vi "PicoScope2000aExampleBlockAdvancedTrigger.vi"() -> ()   [LabVIEW 2010]
doc: "ps2000a API Block Capture example"
uses:
  shared/PicoBuffers.ctl
  <vilib>/Waveform/DWDTOps.llb/DWDT Analog to Digital.vi
  shared/Buffer and Transfer Settings.ctl
  shared/Acquisition Settings.ctl
  PicoScope2000aLib/PicoScope2000aAnalogChannelSettings.ctl
  PicoScope2000aLib/PicoScope2000aDigitalChannelSettings.ctl
panel:
  in  "roundFaster":bool=TRUE
  in  "timeIntervalRequested":dbl format="%#6_6p"
  in  "Write to TDMS":bool
  in  "Pulse Width Qualifier Settings":T1={"Direction"=2, "Lower Limit"=0, "Upper Limit"=0, "Pulse Width Type"=0} {"Pulse Width Type" items=["None", "Less Than", "Greater Than", "In Range", "Out of Range"]; "Direction" items=["Rising"=2, "Falling"=3]}
  in  "Pulse Width Qualifier Conditions":T2 {"Condition Logic" items=["AND", "OR", "XOR"]}
  in  "Auto Trigger (ms)":i32=1000
  in  "Channel A Trigger Properties":T3={"thresholdUpper"=0, "thresholdUpperHysteresis"=0, "thresholdLower"=0, "thresholdLowerHysteresis"=0, "Threshold Mode"=0, "Direction"=0, "Available"=TRUE} {"Direction" items=["Above / Inside", "Below / Outside", "Rising / Enter", "Falling / Exit", "Rising or Falling / Enter or Exit", "Above Lower", "Below Lower", "Rising Lower", "Falling Lower", "Positive Runt", "Negative Runt"]; "Threshold Mode" items=["Level", "Window"]}
  in  "Digital Port  0":T4 {"Direction Channel 7" items=["Don't Care", "Low", "High", "Rising", "Falling"]; "Direction Channel 6" items=["Don't Care", "Low", "High", "Rising", "Falling"]; "Direction Channel 5" items=["Don't Care", "Low", "High", "Rising", "Falling"]; "Direction Channel 4" items=["Don't Care", "Low", "High", "Rising", "Falling"]; "Direction Channel 3" items=["Don't Care", "Low", "High", "Rising", "Falling"]; "Direction Channel 2" items=["Don't Care", "Low", "High", "Rising", "Falling"]; "Direction Channel 1" items=["Don't Care", "Low", "High", "Rising", "Falling"]; "Direction Channel 0" items=["Don't Care", "Low", "High", "Rising", "Falling"]}
  in  "Trigger Conditions":T5 {"Condition Logic" items=["AND", "OR", "XOR"]}
  out "Properties Panel":T6 {"Max Total Capture Time Available (sec)" format="%.3p"; "Sample Frequency" format="%.3p"; "Sample Internal" format="%.3p"; "Max Samples Available" format="%.3p"; "Total Capture Time (sec)" format="%.3p"}
  in  "Port 0 Settings":T7={"Enabled"=FALSE, "Logic Level"=9830} {"Logic Level" items=["1.5V TTL"=9830, "2.5V CMOS"=16383]}
  in  "Channel A Settings":T8={"Enabled"=TRUE, "Coupling"=1, "Range"=6, "Analogue Offset"=0.0} {"Analogue Offset" format="%#_6p"; "Range" items=["20 mV"=1, "50 mV"=2, "100 mV"=3, "200 mV"=4, "500 mV"=5, "1 V"=6, "2 V"=7, "5 V"=8, "10 V"=9, "20 V"=10]; "Coupling" items=["AC", "DC"]}
  out "Device Info":T9={"Driver Version"="2.1.104.3324", "USB Version"="2.0", "Hardware"="1", "Variant"="2206A", "Batch and Serial"="CV676/049", "Cal Date"="19Sep17", "Kernel Version"="1.0", "Digital HW Version"="1", "Analogue HW Version"="1", "Firmware 1"="1.3.3.0", "Firmware 2"="0.5.47.0", "MSO"=FALSE, "Number of Channels"=2}
  out "overflow":i16 format="%06b"
  in  "Apply Settings":bool
  out "error out":errorcluster
  in  "Data file":path=path "PicoScope2000aExampleAdvancedTrgger Data"
  in  "Buffer and Transfer Settings":T10={"startIndex"=0, "Samples"=32000, "Down Sample Ratio"=1, "Down-Sample Mode"=0} {"Down-Sample Mode" items=["RAW none"=2147483648, "None"=0, "Aggregate"=1, "Decimate"=2, "Average"=4]; "Down Sample Ratio" step=1; "Samples" format="%_6p"}
  in  "Acquisition Settings":T11={"preTriggerSamples"=0, "postTriggerSamples"=32000, "timebase"=0} {"postTriggerSamples" format="%_6p"; "preTriggerSamples" format="%_6p"}
  out "Port 0":digitalwaveform(graph)={"t0"=timestamp(0 s since 1904-01-01), "dt"=8e-09, "Y"={"transitions"=[], "data"=[]}}
  in  "stop":bool
  out "Analog Channels":cluster{i32, sgl, "Data":dbl[]}[](graph)
  in  "Serial Number":string
  in  "Use Serial Number":bool
  in  "error in (no error)":errorcluster
  # "Bit 0 = ChA"
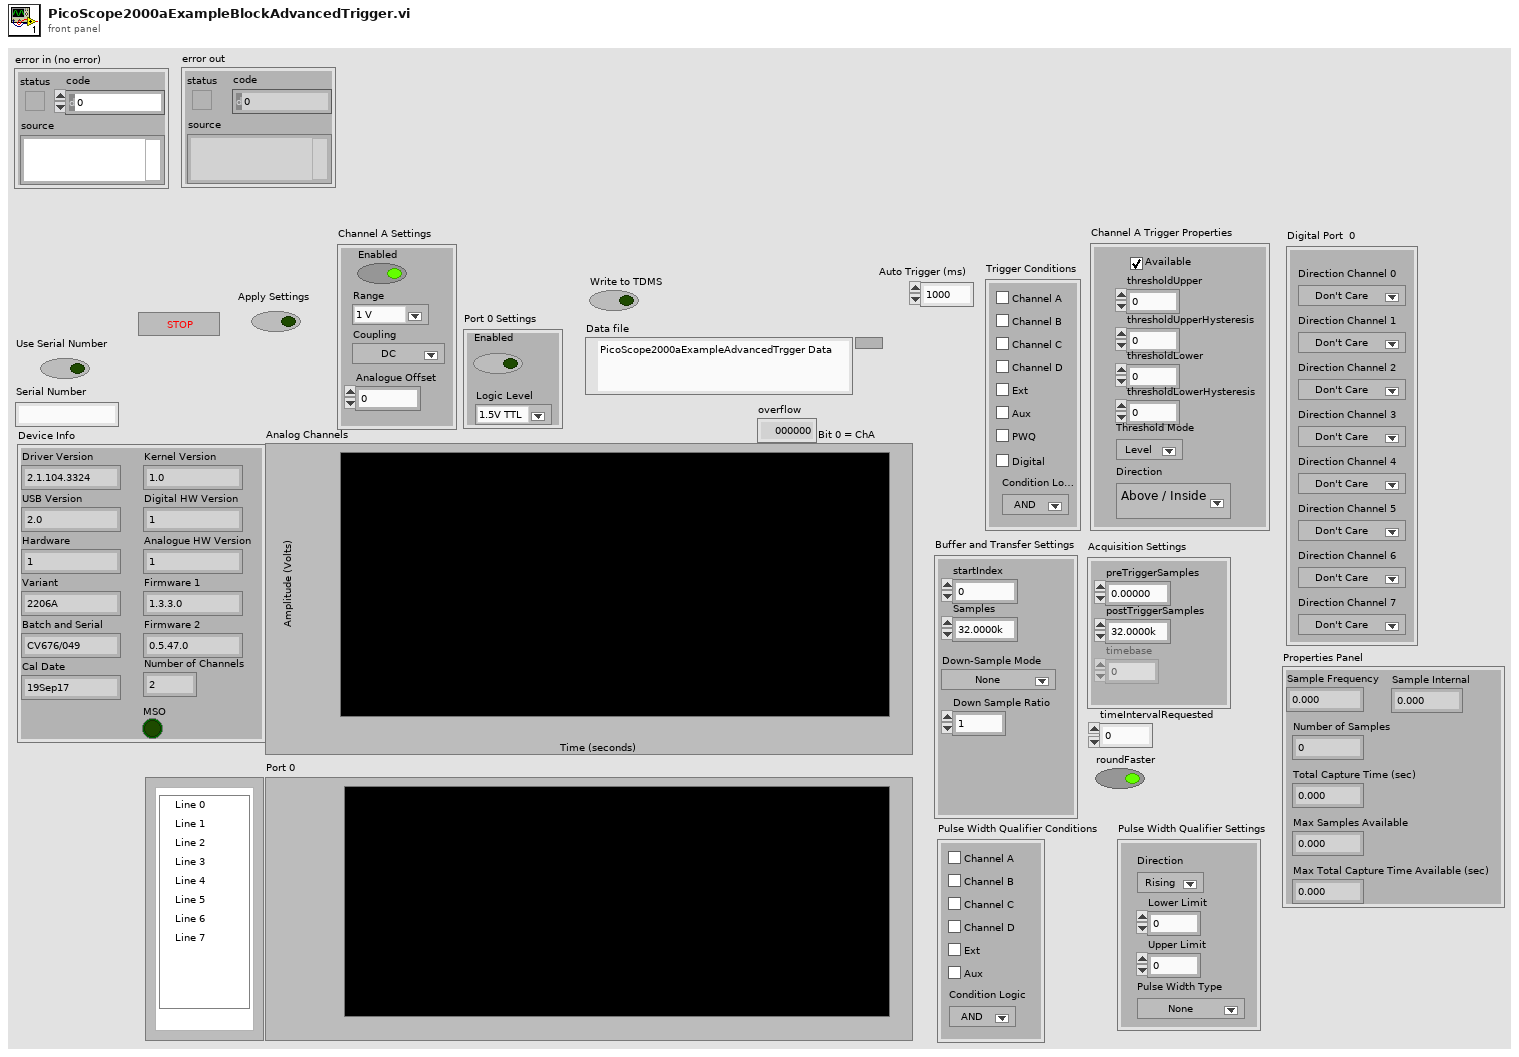
[diagram p1: front panel]
types:
  T1 = cluster{"Direction":i32, "Lower Limit":u32, "Upper Limit":u32, "Pulse Width Type":i32}
  T2 = cluster{"Channel A":bool, "Channel B":bool, "Channel C":bool, "Channel D":bool, "Aux":bool, "Condition Logic":u16, "Ext":bool}
  T3 = cluster{"thresholdUpper":i16, "thresholdUpperHysteresis":u16, "thresholdLower":i16, "thresholdLowerHysteresis":u16, "Threshold Mode":i32, "Direction":i32, "Available":bool}
  T4 = cluster{"Direction Channel 0":u16, "Direction Channel 1":u16, "Direction Channel 2":u16, "Direction Channel 3":u16, "Direction Channel 4":u16, "Direction Channel 5":u16, "Direction Channel 6":u16, "Direction Channel 7":u16}
  T5 = cluster{"Channel A":bool, "Channel B":bool, "Channel C":bool, "Channel D":bool, "Aux":bool, "PWQ":bool, "Condition Logic":u16, "Ext":bool, "Digital":bool}
  T6 = cluster{"Sample Frequency":sgl, "Sample Internal":sgl, "Max Samples Available":i32, "Number of Samples":u32, "Total Capture Time (sec) ":sgl, "Max Total Capture Time Available (sec)":sgl}
  T7 = typedef "PicoScope2000aDigitalChannelSettings.ctl" = cluster{"Enabled":bool, "Logic Level":i16}
  T8 = typedef "PicoScope2000aAnalogChannelSettings.ctl" = cluster{"Enabled":bool, "Coupling":i16, "Range":u32, "Analogue Offset":sgl}
  T9 = cluster{"Driver Version":string, "USB Version":string, "Hardware":string, "Variant":string, "Batch and Serial":string, "Cal Date":string, "Kernel Version":string, "Digital HW Version":string, "Analogue HW Version":string, "Firmware 1":string, "Firmware 2":string, "MSO":bool, "Number of Channels":i16}
  T10 = typedef "Buffer and Transfer Settings.ctl" = cluster{"startIndex":u64, "Samples":u64, "Down Sample Ratio":u64, "Down-Sample Mode":u32}
  T11 = typedef "Acquisition Settings.ctl" = cluster{"preTriggerSamples":u64, "postTriggerSamples":u64, "timebase":u32}
  T12 = typedef "PicoBuffers.ctl" = cluster{"Max Buffer Pointers":u64[][][], "Min Buffer Pointers":u64[][][], "StreamingDataInfo":cluster{"Channel":u32, "Down-Sample Mode":u32, "PICO_DATA_TYPE":enum32{"PICO_INT8_T", "PICO_INT16_T", "PICO_INT32_T", "PICO_UINT32_T", "PICO_INT64_T", ""}, "Samples":i32, "bufferIndex":u64, "startIndex":i32, "overflow":i16}[][]}
  T13 = enum16{"open", "open or create", "create or replace", "create", "open (read-only)"}
  T14 = cluster{"Channel A Buffer":i16[], "Channel B Buffer":i16[], "Channel C Buffer":i16[], "Channel D Buffer":i16[], "Channel E Buffer":i16[], "Channel F Buffer":i16[], "Channel G Buffer":i16[], "Channel H Buffer":i16[], "Port 0 Buffer":i16[], "Port 1 Buffer":i16[]}[]
  T15 = cluster{"Channel A Buffer":i16[], "Channel B Buffer":i16[], "Channel C Buffer":i16[], "Channel D Buffer":i16[], "Channel E Buffer":i16[], "Channel F Buffer":i16[], "Channel G Buffer":i16[], "Channel H Buffer":i16[], "Port 0 Buffer":i16[], "Port 1 Buffer":i16[]}
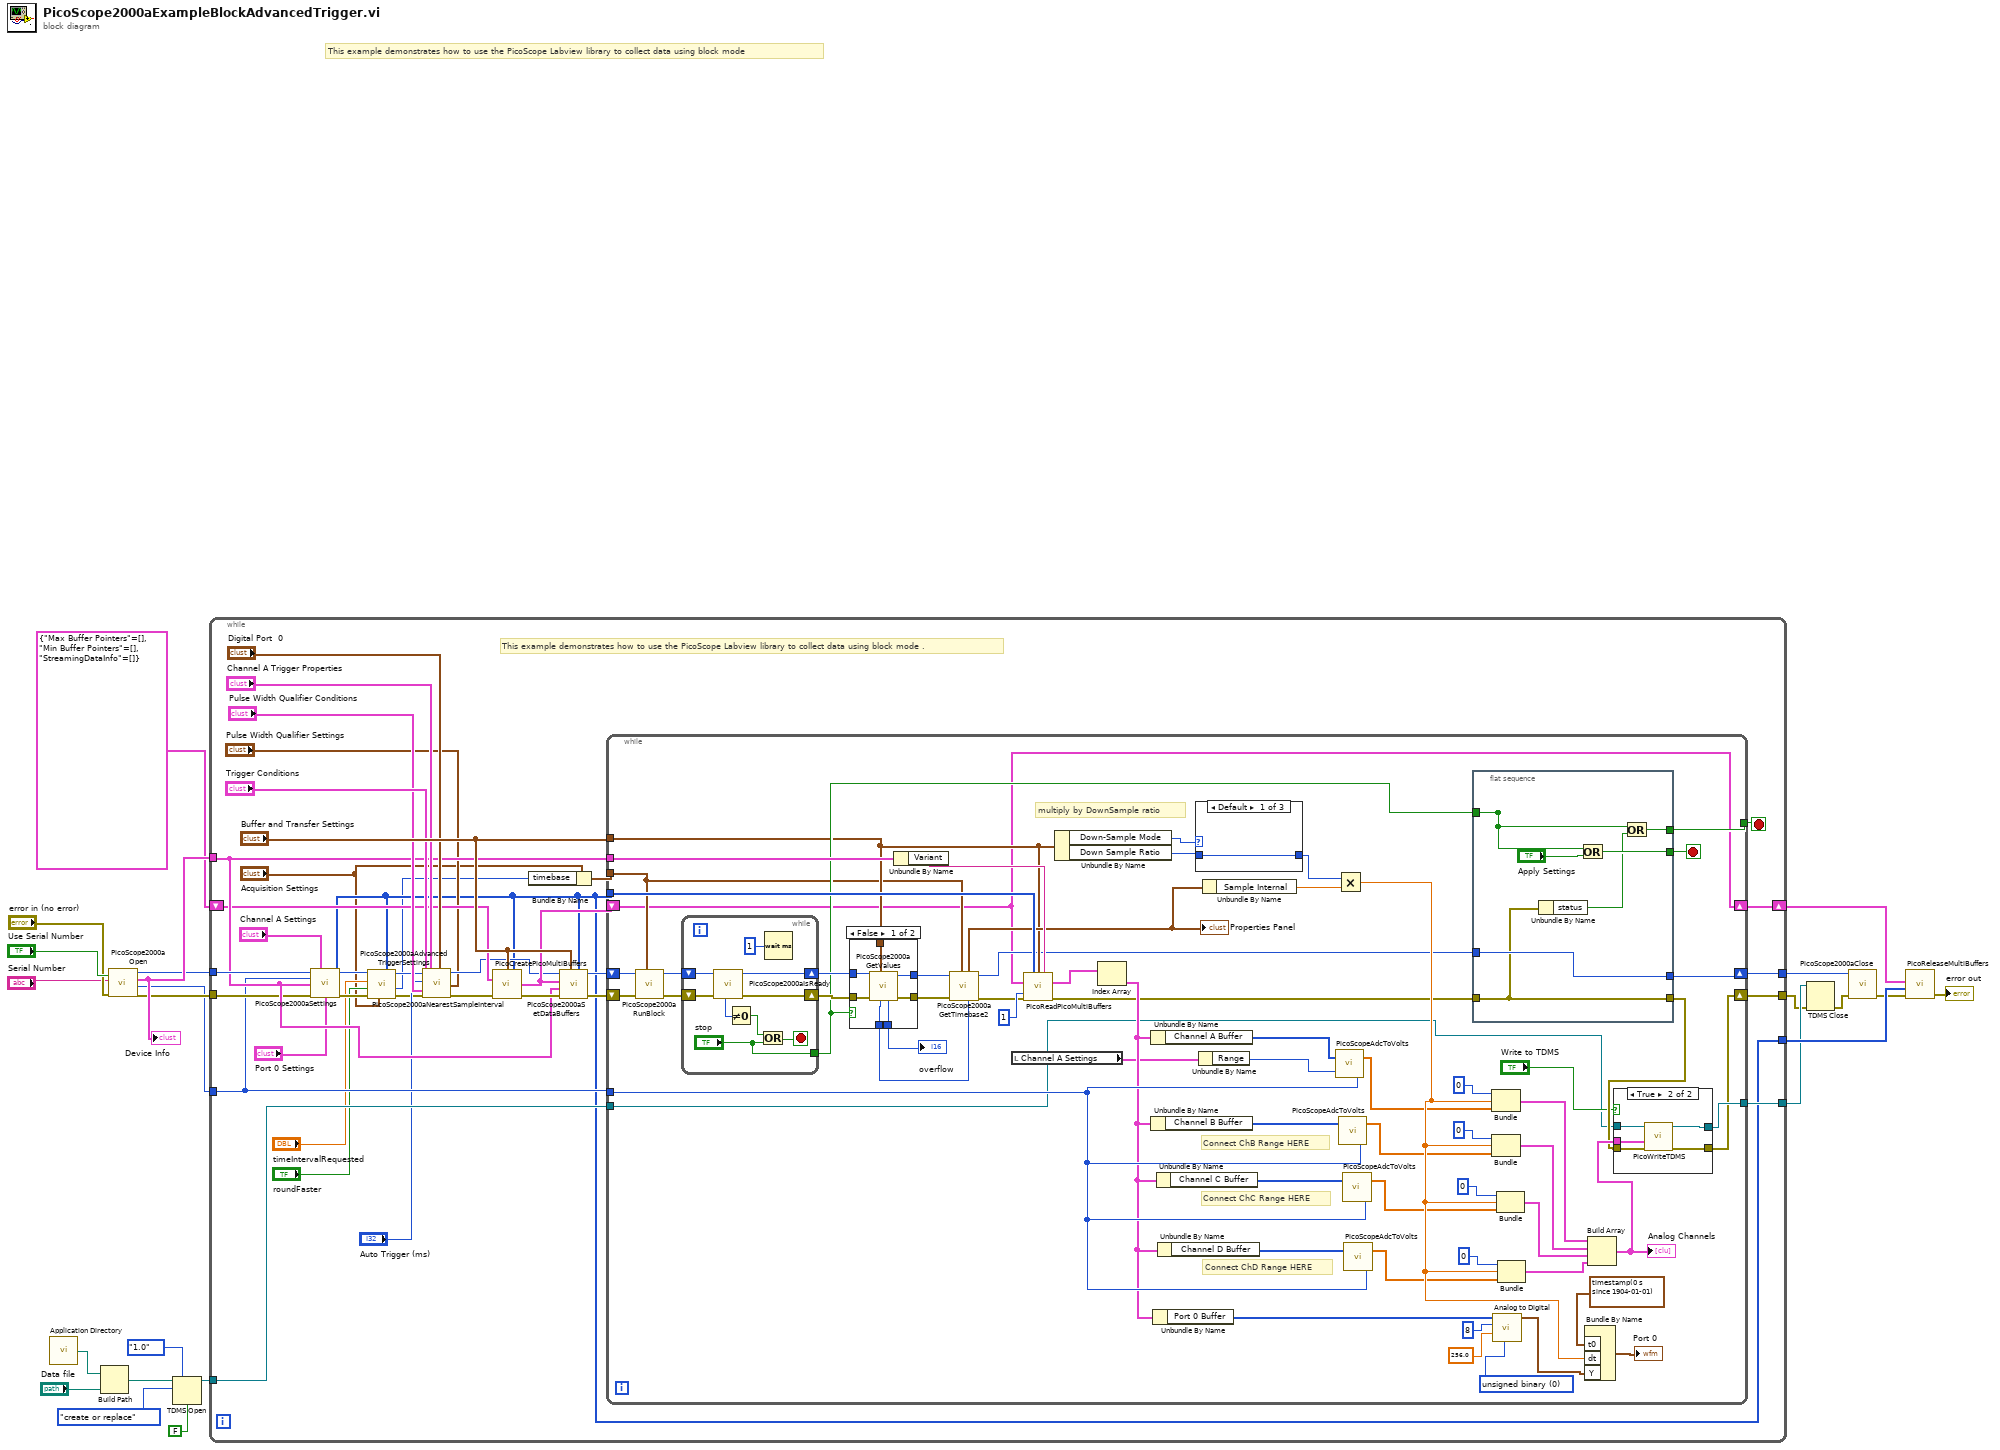
[diagram p0: block diagram]
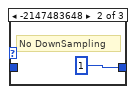
[diagram p4: hidden frame]
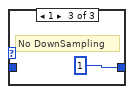
[diagram p5: hidden frame]
diagram:
  # "This example demonstrates how to use the PicoScope Labview library to collect data using block mode"
  n1 = call <vilib>:"Application Directory.vi"() -> ("Application Directory"=w17:path)
  n2 = Build Path(base path=w17, name or relative path="Data file") -> (appended path=w18:path)
  n3 = call "PicoScope2000aOpen.vi"("Serial Number"="Serial Number", "Use Serial Number"="Use Serial Number", "error in (no error)"="error in (no error)") -> ("error out"=w6:errorcluster, "Max Adc value"=w5:i16, "Device Info"=w9:T9, "handle"=w7:i16)  [unwired: 3 in, 2 out]
  "Device Info" <- w9
  n4 = TDMS Open(6:FALSE ("disable buffering? (T)"), 7:enum16{"1.0", "2.0"}."1.0" ("file format version (2.0)"), 10:T13."create or replace" ("operation (0:open)"), 11:w18) -> (3:w15:refnum<k34>)  [unwired: 2 in, 1 out]
  n5 = while {
    tunnel: w5 -> [w41]
    tunnel: [w29] -> w23
    tunnel: [w56] -> w16
    tunnel: w15 -> [w58]
    tunnel: w9 -> [w44]
    tunnel: [w57] -> w2
    tunnel: [w54] -> w10
    tunnel: w7 -> [w45]
    tunnel: w6 -> [w42]
    shift-right: [w38] -> w3
    shift-left: T12 {"Max Buffer Pointers"=[], "Min Buffer Pointers"=[], "StreamingDataInfo"=[]} ("Data Pointers") -> [w40]
    stop <- w55 stop-if-true
    # "This example demonstrates how to use the PicoScope Labview library to collect data using block mode ."
    n6 = call "PicoScope2000aSettings.vi"("handle in"=w45, "Channel A Settings"="Channel A Settings", "Max_adc"=w41, "Device Info"=w44, "error in"=w42, "Port 0 Settings"="Port 0 Settings") -> ("handle out"=w32:i16, "Enabled Array"=w29:i16[], "error out"=w33:errorcluster)  [unwired: 7 in]
    n7 = call "PicoScope2000aNearestSampleInterval.vi"("Enabled array"=w29, "Acquisition Settings"="Acquisition Settings", "error in (no error)"=w33, "roundFaster"="roundFaster", "timeIntervalRequested"="timeIntervalRequested", "handle in"=w32) -> ("error out"=w30:errorcluster, "timebase"=w24:u32, "handle out"=w31:i16)  [unwired: 2 in, 1 out]
    n8 = call "PicoScope2000aAdvancedTriggerSettings.vi"("handle in"=w31, "Auto Trigger (ms)"="Auto Trigger (ms)", "Trigger Conditions"="Trigger Conditions", "error in"=w30, "Channel A Trigger Properties"="Channel A Trigger Properties", "Digital Port  0"="Digital Port  0", "Pulse Width Qualifier Settings"="Pulse Width Qualifier Settings", "Pulse Width Qualifier Conditions"="Pulse Width Qualifier Conditions") -> ("handle out"=w37:i16, "error out"=w36:errorcluster)  [unwired: 10 in]
    n9 = call "PicoCreatePicoMultiBuffers.vi"("Buffer and Transfer Settings"="Buffer and Transfer Settings", "enabled array"=w29, "Data Pointers In"=w40, "error in (no error)"=w36) -> ("Data Pointers"=w39:T12, "error out"=w59:errorcluster)  [unwired: 10 in]
    n10 = Bundle By Name(cluster="Acquisition Settings", "timebase"=w24) -> (w26:T11)
    n11 = call "PicoScope2000aSetDataBuffers.vi"("enabled array"=w29, "Buffer and Transfer Settings"="Buffer and Transfer Settings", "error in (no error)"=w59, "Device Info"=w44, "Data Pointers In"=w39, "handle in"=w37) -> ("error out"=w53:errorcluster, "handle out"=w52:i16)  [unwired: 4 in]
    n12 = while {
      tunnel: "Buffer and Transfer Settings" -> [w73]
      tunnel: w29 -> [w116]
      tunnel: w26 -> [w72]
      tunnel: w41 -> [w115]
      tunnel: w44 -> [w112]
      tunnel: [w84] -> w55
      shift-right: [w64] -> w57
      shift-left: w53 -> [w78]
      shift-right: [w82] -> w54
      shift-left: w52 -> [w79]
      tunnel: w58 -> [w61]
      tunnel: [w67] -> w56
      shift-right: [w63] -> w38
      shift-left: w39 -> [w63]
      stop <- w83 stop-if-true
      w102 = u16 0 items=["unsigned binary", "offset binary", "2's complement"] ("data format (offset binary)")
      # "Connect ChB Range HERE"
      # "Connect ChD Range HERE"
      # "Connect ChC Range HERE"
      # "multiply by DownSample ratio"
      n13 = call "PicoScope2000aRunBlock.vi"("Acquisition Settings"=w72, "error in (no error)"=w78, "handle in"=w79) -> ("error out"=w118:errorcluster, "handle out"=w117:i16)  [unwired: 5 in, 2 out]
      n14 = while {
        shift-right: [w154] -> w80
        shift-left: w118 -> [w155]
        shift-right: [w153] -> w81
        shift-left: w117 -> [w152]
        tunnel: ["stop"] -> w77
        stop <- w149 stop-if-true
        n15 = call "PicoScope2000aIsReady.vi"("error in (no error)"=w155, "handle in"=w152) -> ("error out"=w154:errorcluster, "handle out"=w153:i16, "ready"=w151:i16)  [unwired: 7 in]
        n16 = Not Equal To 0?(x=w151) -> (x != 0?=w150:bool)
        n17 = Or(x=w150, y="stop") -> (x .or. y?=w149:bool)
        n18 = Wait (ms)(milliseconds to wait=u32 1) -> ()  [unwired: 1 out]
      }
      n19 = case shown="False" w77 {
        tunnel: w80 -> [w137 w138]
        tunnel: w81 -> [w136 w139]
        tunnel: [w135 w139] -> w70
        tunnel: [w134 w138] -> w71
        tunnel: w73 -> [w133 _]
        tunnel: [w132 _] -> w76
        tunnel: [w131 _] -> w75
        frame False {
          n20 = call "PicoScope2000aGetValues.vi"("Buffer and Transfer Settings"=w133, "error in (no error)"=w137, "handle in"=w136) -> ("error out"=w134:errorcluster, "handle out"=w135:i16, "overflow"=w132:i16, "noOfSamples"=w131:u64)  [unwired: 5 in]
        }
        frame True {
        }
      }
      "overflow" <- w76
      n21 = Unbundle By Name(w112) -> ("Variant"=w113:string)
      n22 = call "PicoScope2000aGetTimebase2.vi"("Number of Samples"=w75, "Acquisition Settings"=w72, "error in (no error)"=w71, "handle in"=w70) -> ("error out"=w69:errorcluster, "handle out"=w68:i16, "Properties Panel"=w74:T6)  [unwired: 5 in]
      "Properties Panel" <- w74
      n23 = local read "Channel A Settings"() -> (w60:T8)
      n24 = call "PicoReadPicoMultiBuffers.vi"("enabled array"=w116, "Buffer and Transfer Settings"=w73, "Variant"=w113, "Data Pointers"=w63, "No of Buffers"=1, "error in (no error)"=w69) -> ("MultiBuffers (Max or non-aggregated)"=w123:T14, "error out"=w85:errorcluster)  [unwired: 7 in, 1 out]
      n25 = Unbundle By Name(w73) -> ("Down-Sample Mode"=w121:u32, "Down Sample Ratio"=w122:u64)
      n26 = Index Array(array=w123) -> (element=w86:T15)  [unwired: 1 in]
      n27 = Unbundle By Name(w86) -> ("Channel A Buffer"=w95:i16[])
      n28 = Unbundle By Name(w86) -> ("Channel B Buffer"=w107:i16[])
      n29 = Unbundle By Name(w86) -> ("Port 0 Buffer"=w100:i16[])
      n30 = Unbundle By Name(w86) -> ("Channel C Buffer"=w93:i16[])
      n31 = Unbundle By Name(w86) -> ("Channel D Buffer"=w89:i16[])
      n32 = case shown="Default" w121 {
        tunnel: [w156 u64 1 ("Down Sample Ratio") u64 1 ("Down Sample Ratio")] -> w119
        tunnel: w122 -> [w156 _ _]
        frame Default {
        }
        frame -2147483648 {
          # "No DownSampling"
        }
        frame 1 {
          # "No DownSampling"
        }
      }
      n33 = Unbundle By Name(w60) -> ("Range"=w109:u32)
      n34 = Unbundle By Name(w74) -> ("Sample Internal"=w114:sgl)
      n35 = call "PicoScopeAdcToVolts.vi"("Max_adc"=w115, "Range Index"=w109, "Data"=w95) -> ("Data"=w96:dbl[])
      n36 = Multiply(x=w119, y=w114) -> (x*y=w120:sgl)
      n37 = call "PicoScopeAdcToVolts.vi"("Max_adc"=w115, "Data"=w107) -> ("Data"=w106:dbl[])  [unwired: 1 in]
      n38 = call "PicoScopeAdcToVolts.vi"("Max_adc"=w115, "Data"=w93) -> ("Data"=w92:dbl[])  [unwired: 1 in]
      n39 = call "PicoScopeAdcToVolts.vi"("Max_adc"=w115, "Data"=w89) -> ("Data"=w88:dbl[])  [unwired: 1 in]
      n40 = flat-sequence {
        tunnel: [w146] -> w83
        tunnel: [w140] -> _
        tunnel: [w143] -> w84
        tunnel: w68 -> [w142]
        tunnel: [w142] -> w82
        tunnel: w85 -> [w141]
        tunnel: [w141] -> w65
        tunnel: w77 -> [w140]
        frame #0 {
          n41 = Unbundle By Name(w141) -> ("status"=w144:bool)
          n42 = Or(x=w140, y="Apply Settings") -> (x .or. y?=w146:bool)
          n43 = Or(x=w140, y=w144) -> (x .or. y?=w143:bool)
        }
      }
      n44 = Bundle(0, w120, "Data"=w96) -> (w105:cluster{i32, sgl, "Data":dbl[]})  [unwired: 1 in]
      n45 = Bundle(0, w120, "Data"=w106) -> (w104:cluster{i32, sgl, "Data":dbl[]})  [unwired: 1 in]
      n46 = call-poly <vilib>:"Analog to Digital.vi"("data format (offset binary)"=w102, "full-scale range (pk-pk)"=256.0, "resolution (16 bit)"=8, "analog waveform"=w100) -> ("digital waveform"=w97:digitalwaveform)  [unwired: 4 in, 3 out]
      n47 = Bundle(0, w120, "Data"=w92) -> (w91:cluster{i32, sgl, "Data":dbl[]})  [unwired: 1 in]
      n48 = Bundle(0, w120, "Data"=w88) -> (w87:cluster{i32, sgl, "Data":dbl[]})  [unwired: 1 in]
      n49 = Bundle By Name("t0"=timestamp(0 s since 1904-01-01), "dt"=w120, "Y"=w97) -> (→"Port 0":digitalwaveform)  [unwired: 1 in]
      n50 = Build Array(w105, w104, w91, w87) -> (w66:cluster{i32, sgl, "Data":dbl[]}[])
      "Analog Channels" <- w66
      n51 = case shown="True" "Write to TDMS" {
        tunnel: w66 -> [_ w130]
        tunnel: w61 -> [w124 w129]
        tunnel: w65 -> [w125 w128]
        tunnel: [w125 w127] -> w64
        tunnel: [w124 w126] -> w67
        frame False {
        }
        frame True {
          n52 = call "PicoWriteTDMS.vi"("error in (no error)"=w128, "Analog Channels"=w130, "Refnum in"=w129) -> ("error out"=w127:errorcluster, "Refnum out"=w126:refnum<k34>)  [unwired: 7 in]
        }
      }
    }
  }
  n53 = TDMS Close(8:w2, 11:w16) -> (0:w1:errorcluster)  [unwired: 1 out]
  n54 = call "PicoScope2000aClose.vi"("error in (no error)"=w1, "handle in"=w10) -> ("error out"=w8:errorcluster)  [unwired: 8 in, 1 out]
  n55 = call "PicoReleaseMultiBuffers.vi"("error in (no error)"=w8, "Enabled array"=w23, "Data Pointers"=w3) -> ("error out"=→"error out":errorcluster)  [unwired: 7 in, 1 out]
